vi "Deserialize_NonBlueObject.vi"(8 "error in (no error)":errorcluster, 9 "StructuredData in":variant, 10 "Object Type":refnum<class>, 11 "BlueSerializer in":refnum<class "BlueSerializer.lvclass">) -> (0 "error out":errorcluster, 1 "StructuredData out":variant, 2 "Object out":refnum<class>, 3 "BlueSerializer out":refnum<class "BlueSerializer.lvclass">)   [LabVIEW 2019, in "BlueSerialization.lvlib" / "BlueSerializer.lvclass"]
uses:
  BlueSerializer.lvclass
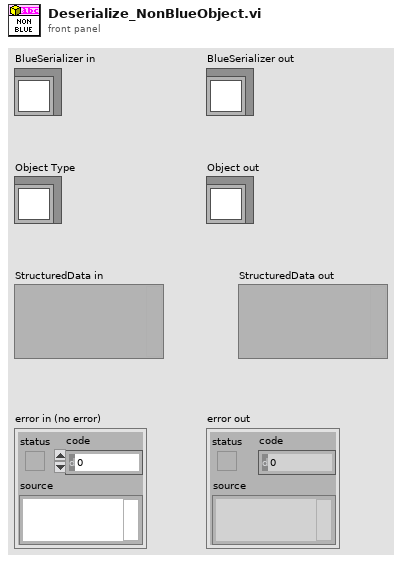
[diagram p1: front panel]
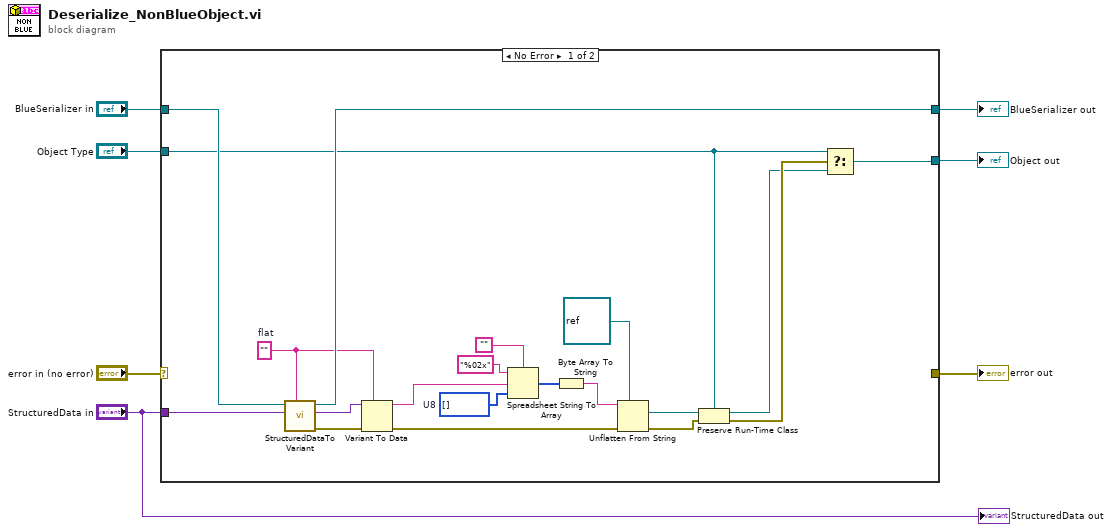
[diagram p0: block diagram]
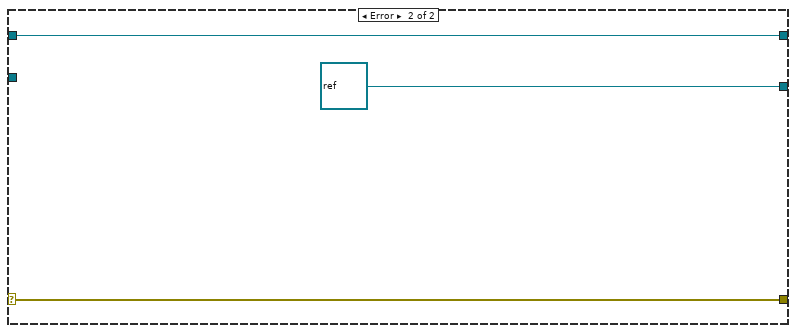
[diagram p2: hidden frame]
diagram:
  n1 = case shown="No Error" "error in (no error)" {
    selector: "error in (no error)" -> [_ w30]
    tunnel: "BlueSerializer in" -> [w27 w29]
    tunnel: [w26 w29] -> w6
    tunnel: "Object Type" -> [w25 _]
    tunnel: "StructuredData in" -> [w24 _]
    tunnel: [w23 refnum<class> refnum ("Object Type")] -> w4
    tunnel: [_ w30] -> w2
    frame No Error {
      w13 = u8[] []  # U8
      w15 = ""  # flat
      n2 = call-dynamic "StructuredDataToVariant.vi"("Data Type"=w15, "StructuredData"=w24, "BlueSerializer in"=w27) -> ("error out"=w16:errorcluster, "Variant"=w17:variant, "BlueSerializer out"=w26:refnum<class "BlueSerializer.lvclass">)  [unwired: 6 in]
      n3 = Variant To Data(error in=w16, type=w15, Variant=w17) -> (data=w10:string, error out=w8:errorcluster)
      n4 = Spreadsheet String To Array(delimiter (Tab)="", format string="%02x", spreadsheet string=w10, array type (2D Dbl)=w13) -> (array=w14:u8[])
      n5 = Byte Array To String(unsigned byte array=w14) -> (string=w9:string)
      n6 = Unflatten From String(type=refnum<class> refnum ("LabVIEW Object"), binary string=w9, error in (no error)=w8) -> (value=w22:refnum<class>, error out=w21:errorcluster)  [unwired: 2 in, 1 out]
      n7 = Preserve Run-Time Class(object in=w22, error in=w21, 2:w25) -> (object out=w19:refnum<class>, error out=w20:errorcluster)
      n8 = Select(t=w25, s=w20, f=w19) -> (s? t:f=w23:refnum<class>)
    }
    frame Error {
    }
  }
  "error out" <- w2
  "BlueSerializer out" <- w6
  "Object out" <- w4
  "StructuredData out" <- "StructuredData in"
